vi "insertScriptEventIntoDevice.vi"(8 "error in (no error)":errorcluster, 10 "ScriptEvent":refnum<class "ScriptEvent.lvclass">, 11 "DeviceArray in":refnum<class "DeviceArray.lvclass">) -> (0 "error out":errorcluster, 3 "DeviceArray out":refnum<class "DeviceArray.lvclass">)   [LabVIEW 2011, in "Tools.lvlib" / "DatabaseHelpers.lvlib" / "DeviceArray.lvclass"]
uses:
  DeviceArray.lvclass
  Scripting/ScriptingEvent/ScriptEvent.lvclass
  Channel/Channel.lvclass
  device/device.lvclass
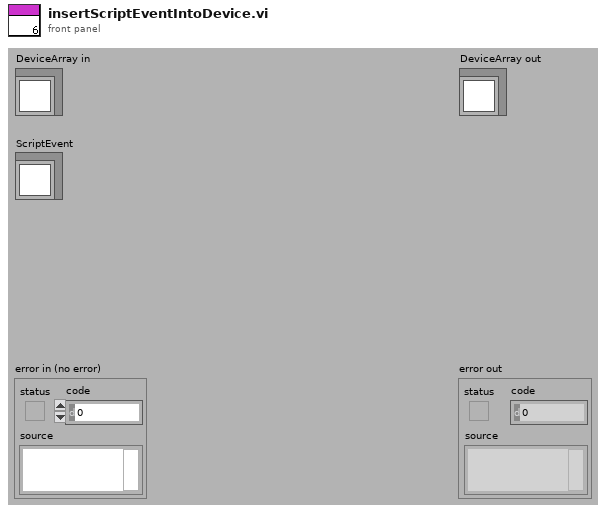
[diagram p1: front panel]
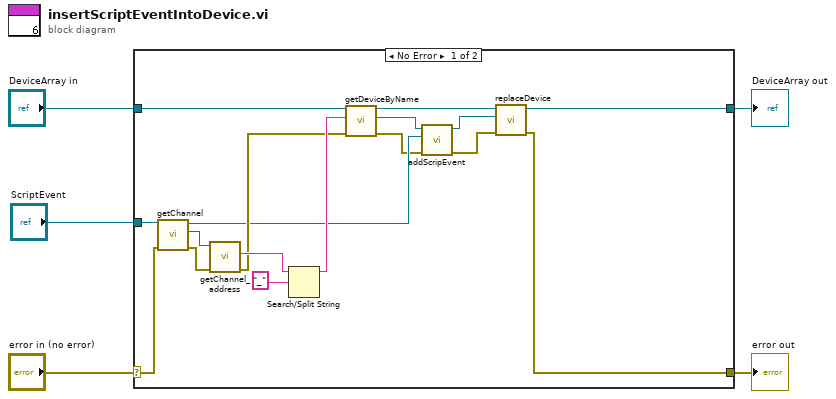
[diagram p0: block diagram]
diagram:
  n1 = case shown="No Error" "error in (no error)" {
    selector: "error in (no error)" -> [w14 w24]
    tunnel: [w6 w24] -> w4
    tunnel: [w7 w23] -> w2
    tunnel: "DeviceArray in" -> [w20 w23]
    tunnel: "ScriptEvent" -> [w13 _]
    frame No Error {
      n2 = call-dynamic "getChannel.vi"("error in (no error)"=w14, "ScriptEvent.lvclass in"=w13) -> ("error out"=w15:errorcluster, "Channel.lvclass"=w16:refnum<class "Channel.lvclass">, "ScriptEvent.lvclass out"=w12:refnum<class "ScriptEvent.lvclass">)  [unwired: 7 in]
      n3 = call "getChannel_address.vi"("error in (no error)"=w15, "Channel.lvclass in"=w16) -> ("error out"=w18:errorcluster, "channel_address"=w22:string)  [unwired: 7 in, 1 out]
      n4 = Search/Split String(string=w22, search string/char (-)="_") -> (substring before match=w19:string)  [unwired: 1 in, 2 out]
      n5 = call "getDeviceByName.vi"("error in (no error)"=w18, "deviceName"=w19, "DeviceArray in"=w20) -> ("error out"=w11:errorcluster, "device.lvclass"=w17:refnum<class "device.lvclass">, "DeviceArray out"=w10:refnum<class "DeviceArray.lvclass">)  [unwired: 5 in, 1 out]
      n6 = call "addScripEvent.vi"("error in (no error)"=w11, "ScriptEvent"=w12, "device in"=w17) -> ("error out"=w8:errorcluster, "device out"=w9:refnum<class "device.lvclass">)  [unwired: 7 in]
      n7 = call "replaceDevice.vi"("error in (no error)"=w8, "device"=w9, "DeviceArray in"=w10) -> ("error out"=w6:errorcluster, "DeviceArray out"=w7:refnum<class "DeviceArray.lvclass">)  [unwired: 7 in]
    }
    frame Error {
    }
  }
  "error out" <- w4
  "DeviceArray out" <- w2
